vi "Get register for reading - array.vi"(11 "Reg array in":string[](array[string])) -> (3 "Reg array out":string[](array[string]))   [LabVIEW 2020, in "Toggle 8.lvclass"]
uses:
  Toggle 8.lvclass
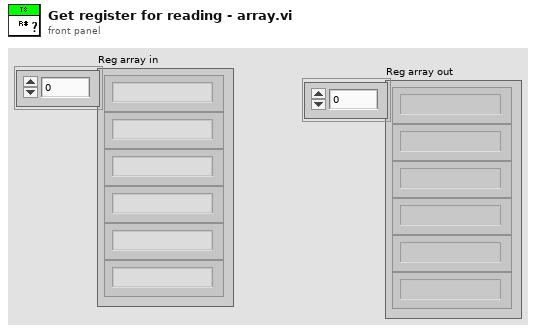
[diagram p1: front panel]
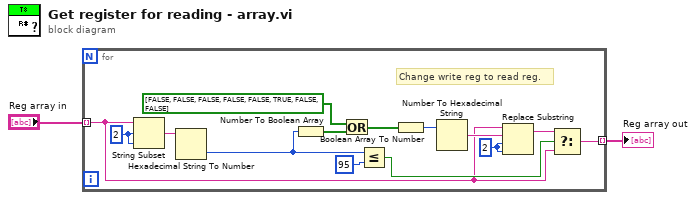
[diagram p0: block diagram]
diagram:
  n1 = for {
    tunnel: "Reg array in" -> [w4] mode=indexing
    tunnel: [w3] -> w1 mode=indexing
    w10 = 2 ("offset (0)")
    w9 = 2 ("length (rest)")
    # "Change write reg to read reg."
    n2 = String Subset(string=w4, offset (0)=w9, length (rest)=w9) -> (substring=w12:string)
    n3 = Hexadecimal String To Number(string=w12) -> (number=w8:u32)  [unwired: 2 in, 1 out]
    n4 = Number To Boolean Array(number=w8) -> (Boolean array=w15:bool[])
    n5 = Or(x=bool[] [FALSE, FALSE, FALSE, FALSE, FALSE, TRUE, FALSE, FALSE] ("Boolean array"), y=w15) -> (x .or. y?=w14:bool[])
    n6 = Less Or Equal?(x=w8, y=u32 95) -> (x <= y?=w6:bool)
    n7 = Boolean Array To Number(Boolean array=w14) -> (number=w13:u32)
    n8 = Number To Hexadecimal String(2:w13) -> (0:w11:string)  [unwired: 1 in]
    n9 = Replace Substring(2:w10, 3:w10, 4:w11, 5:w4) -> (1:w5:string)  [unwired: 1 out]
    n10 = Select(t=w5, s=w6, f=w4) -> (s? t:f=w3:string)
  }
  "Reg array out" <- w1
